vi "segment_size.vi"() -> ()   [LabVIEW 2013]
panel:
  out "sgmt_size":i32=1000
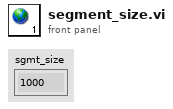
[diagram p1: front panel]
diagram:
